vi "time_conv.vi"() -> ()   [LabVIEW 2023]
panel:
  out "SECONDS":dbl
  out "MINUTES":dbl
  out "HOURS":dbl
  in  "SECONDS":dbl
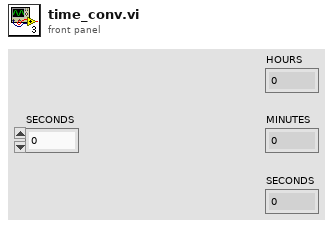
[diagram p1: front panel]
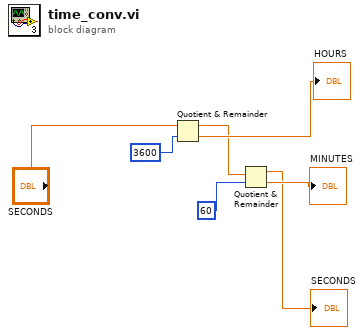
[diagram p0: block diagram]
diagram:
  n1 = Quotient & Remainder(x="SECONDS", y=3600) -> (x-y*floor(x/y)=w2:dbl, floor(x/y)=→"HOURS":dbl)
  n2 = Quotient & Remainder(x=w2, y=60) -> (x-y*floor(x/y)=→"SECONDS":dbl, floor(x/y)=→"MINUTES":dbl)
